vi "Update Occupied Area.vi"(8 "error in (no error)":errorcluster, 11 "UI Controller in":refnum<class "UI Controller.lvclass">) -> (0 "error out":errorcluster, 3 "UI Controller out":refnum<class "UI Controller.lvclass">)   [LabVIEW 2020, in "UI Controller.lvlib" / "UI Controller.lvclass"]
uses:
  UI Controller.lvclass
  C:/Program Files/National Instruments/LabVIEW 2020/vi.lib/ActorFrameworkMVC/View Controller/View Controller/View Controller.lvclass
  UI Controller.lvclass/UI Controller.ctl
  <vilib>/ActorFrameworkMVC/View Controller/View Controller/View Controller.lvclass
panel:
  # "NOTICE -- YOU MUST LEAVE THIS NOTICE IN PLACE.\n\nCopyright (c) 2017, LIANG LIU Shawn.Liu.cn@gmail.com\nAll rights reserved.\n\nRedistribution and use in source and binary forms, with or without modification, are permitted provided that the following conditions are met:\n-Redistributions of source code must retain the above copyright notice, this list of conditions and the following disclaimer.\n-Redistributions in binary form must reproduce the above copyright notice, this list of conditions and the following disclaimer in the documentation and/or other materials provided with the distribution.\n-Neither the name of the eLp nor the names of its contributors may be used to endorse or promote products derived from this software without specific prior written permission.\n\nTHIS SOFTWARE IS PROVIDED BY THE COPYRIGHT HOLDERS AND CONTRIBUTORS \"AS IS\" AND ANY EXPRESS OR IMPLIED WARRANTIES, INCLUDING, BUT NOT LIMITED TO, THE IMPLIED WARRANTIES OF MERCHANTABILITY AND FITNESS FOR A PARTICULAR PURPOSE ARE DISCLAIMED. IN NO EVENT SHALL THE COPYRIGHT HOLDER OR CONTRIBUTORS BE LIABLE FOR ANY DIRECT, INDIRECT, INCIDENTAL, SPECIAL, EXEMPLARY, OR CONSEQUENTIAL DAMAGES (INCLUDING, BUT NOT LIMITED TO, PROCUREMENT OF SUBSTITUTE GOODS OR SERVICES; LOSS OF USE, DATA, OR PROFITS; OR BUSINESS INTERRUPTION) HOWEVER CAUSED AND ON ANY THEORY OF LIABILITY, WHETHER IN CONTRACT, STRICT LIABILITY, OR TORT (INCLUDING NEGLIGENCE OR OTHERWISE) ARISING IN ANY WAY OUT OF THE USE OF THIS SOFTWARE, EVEN IF ADVISED OF THE POSSIBILITY OF SUCH DAMAGE."
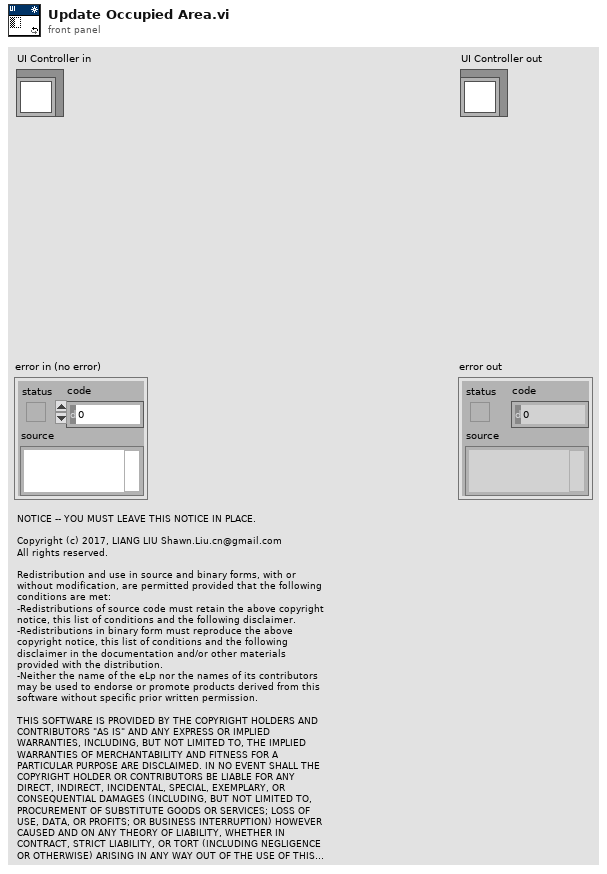
[diagram p1: front panel]
types:
  T1 = cluster{"Left":i16, "Top":i16, "Right":i16, "Bottom":i16}
  T2 = typedef "LVRectTypeDef.ctl" = cluster{"Left":i16, "Top":i16, "Right":i16, "Bottom":i16}
  T3 = cluster{"left":i16, "top":i16, "right":i16, "bottom":i16}
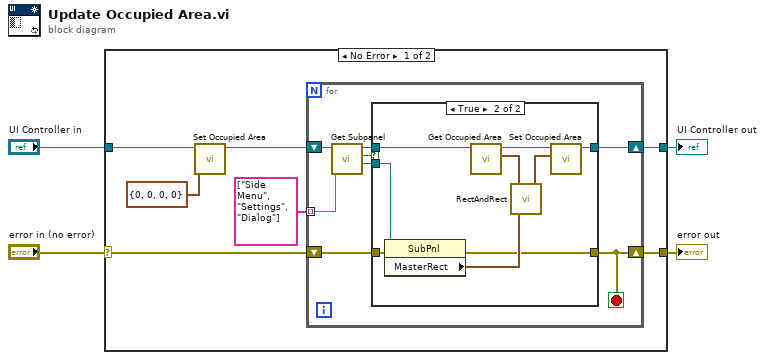
[diagram p0: block diagram]
diagram:
  n1 = case shown="No Error" "error in (no error)" {
    selector: "error in (no error)" -> [w9 w32]
    tunnel: "UI Controller in" -> [w11 w31]
    tunnel: [w10 w31] -> w3
    tunnel: [w8 w32] -> w1
    frame No Error {
      n2 = call "Set Occupied Area.vi"("Occupied Area"=T1 {"Left"=0, "Top"=0, "Right"=0, "Bottom"=0}, "UI Controller in"=w11) -> ("UI Controller out"=w6:refnum<class "UI Controller.lvclass">)  [unwired: 9 in]
      n3 = for {
        shift-right: [w14] -> w10
        shift-left: w6 -> [w19]
        tunnel: string[] ["Side Menu", "Settings", "Dialog"] -> [w18] mode=indexing
        shift-right: [w12] -> w8
        shift-left: w9 -> [w13]
        stop <- w12 stop-if-true
        n4 = call <vilib>:"Get Subpanel.vi"("Subpanel Name"=w18, "View Controller in"=w19) -> ("Subpanel Reference"=w16:refnum<vi>, "Found?"=w17:bool, "View Controller out"=w15:refnum<class "UI Controller.lvclass">)  [unwired: 6 in, 1 out]
        n5 = case shown="True" w17 {
          tunnel: w16 -> [_ w30]
          tunnel: w15 -> [w21 w29]
          tunnel: [w21 w27] -> w14
          tunnel: w13 -> [w20 w23]
          tunnel: [w20 w22] -> w12
          frame False {
          }
          frame True {
            n6 = property class="SubPnl"(reference=w30, error in=w23) -> (error out=w22:errorcluster, "MasterRect"=w26:T2)  [unwired: 1 out]
            n7 = call "Get Occupied Area.vi"("UI Controller in"=w29) -> ("Occupied Area"=w24:T1, "UI Controller out"=w28:refnum<class "UI Controller.lvclass">)  [unwired: 9 in]
            n8 = call <vilib>:"RectAndRect.vi"("rect b"=w26, "rect a"=w24) -> ("union rect"=w25:T3)
            n9 = call "Set Occupied Area.vi"("Occupied Area"=w25, "UI Controller in"=w28) -> ("UI Controller out"=w27:refnum<class "UI Controller.lvclass">)  [unwired: 9 in]
          }
        }
      }
    }
    frame Error {
    }
  }
  "error out" <- w1
  "UI Controller out" <- w3
